vi "FLiNaK Characteristics.vi"(9 "Sec Cold Temp (K)":dbl, 10 "Sec Hot Temp (K)":dbl, 11 "Sec Ave Temp (K)":dbl) -> (0 "Sec Ave Density (kg/m^3) 3":dbl, 1 "Sec Hot Density (kg/m^3) 2":dbl, 2 "Sec Cold Density (kg/m^3)":dbl, 4 "FLiNaK Cold Viscosity (Pa-s)":dbl, 5 "Cp of FLiNaK (J/kgK)":dbl, 6 "FLiNaK Hot Viscosity (Pa-s)":dbl, 8 "FLiNaK Ave Viscosity (Pa-s)":dbl)   [LabVIEW 2019]
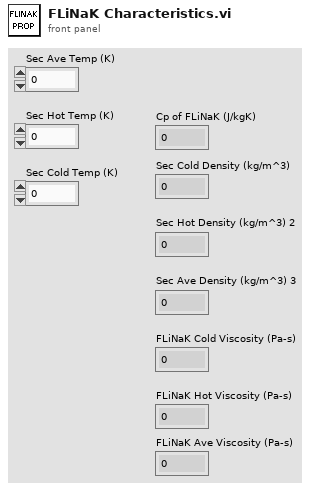
[diagram p1: front panel]
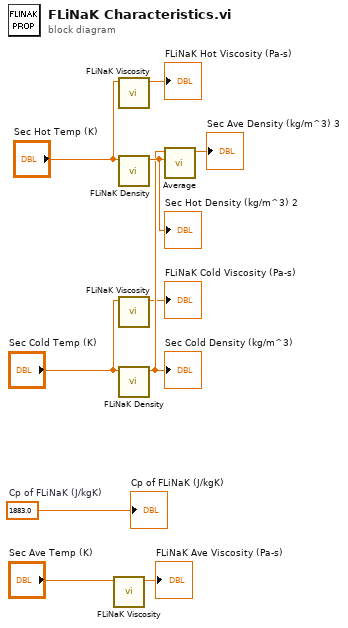
[diagram p0: block diagram]
diagram:
  w1 = 1883.0  # Cp of FLiNaK (J/kgK)
  n1 = call "FLiNaK Viscosity.vi"("Temperature (K)"="Sec Ave Temp (K)") -> ("FLiNaK Viscosity (Pa-s)"=→"FLiNaK Ave Viscosity (Pa-s)":dbl)  [unwired: 10 in]
  n2 = call "FLiNaK Viscosity.vi"("Temperature (K)"="Sec Hot Temp (K)") -> ("FLiNaK Viscosity (Pa-s)"=→"FLiNaK Hot Viscosity (Pa-s)":dbl)  [unwired: 10 in]
  n3 = call "FLiNaK Density.vi"("FLiNaK Temp (K)"="Sec Hot Temp (K)") -> ("FLiNaK Density (kg/m^3)"=w9:dbl)  [unwired: 10 in]
  "Sec Hot Density (kg/m^3) 2" <- w9
  n4 = call "FLiNaK Viscosity.vi"("Temperature (K)"="Sec Cold Temp (K)") -> ("FLiNaK Viscosity (Pa-s)"=→"FLiNaK Cold Viscosity (Pa-s)":dbl)  [unwired: 10 in]
  n5 = call "FLiNaK Density.vi"("FLiNaK Temp (K)"="Sec Cold Temp (K)") -> ("FLiNaK Density (kg/m^3)"=w8:dbl)  [unwired: 10 in]
  "Sec Cold Density (kg/m^3)" <- w8
  n6 = call "Average.vi"("Number 2"=w9, "Number 1"=w8) -> ("Average"=→"Sec Ave Density (kg/m^3) 3":dbl)  [unwired: 9 in]
  "Cp of FLiNaK (J/kgK)" <- w1
